vi "Periodic Tasks.vi"(8 "error in":errorcluster) -> ()   [LabVIEW 2020]
doc: "This VI runs in parallel to other tasks. It can contain as many user-defined periodic loops as you need. These can carry out PID or other sorts of timed response."
uses:
  <vilib>/Rock Robotics/WPI/Utilities/WPI_GetSetVariantRefNum.vi
  Robot Global Data.vi
panel:
  out "Limit Switch":bool
  out "Inverted 4":bool
  out "Inverted 3":bool
  out "Inverted 2":bool
  out "Inverted":bool
  out "Right High":dbl
  out "Left High":dbl
  out "Right Low":dbl format="%#_6f"
  out "Left Low":dbl
  out "Arm Red":dbl
  out "Arm Blue2":dbl
  out "Arm Blue":dbl
  out "Fused Heading":dbl
  out "Heading":dbl
  out "Pitch":dbl
  out "Roll":dbl
  out "Calculated yaw":dbl
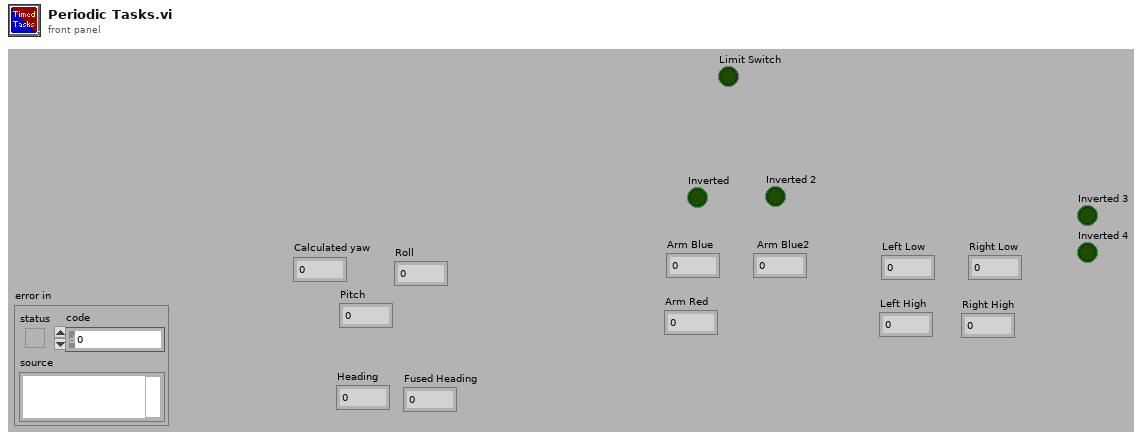
[diagram p1: front panel]
types:
  T1 = typedef "WPI_RobotDriveDevRef.ctl" = cluster{"DevStatus":errorcluster, "Motors[]":T2[], "Square Inputs":bool, "Max Output":dbl}
  T2 = typedef "WPI_MotorControlDeviceRef.ctl" = cluster{"DeviceStatus":errorcluster, "Type":T3, "PWM":cluster{"PWM Channel":T4, "DeadBand":T5}, "CAN":cluster{"Device Number":u8, "SetOutput VI Ref":variant, "GetOutput VI Ref":variant, "Enable VI Ref":variant, "Disable VI Ref":variant, "Data":variant}, "Invert":bool, "DIO PWM":cluster{"PWM \"Enable\" Channel":T4, "DIOChannel":T6, "PWM Rate":dbl}}
  T3 = typedef "WPI_MotorControlType.ctl" = enum16{"PWM", "CAN", "DIO PWM"}
  T4 = typedef "FPGA_DIOPWMChannel.ctl" = enum8{"PWM 0", "PWM 1", "PWM 2", "PWM 3", "PWM 4", "PWM 5", "PWM 6", "PWM 7", "PWM 8", "PWM 9", "PWM MXP 0", "PWM MXP 1", "PWM MXP 2", "PWM MXP 3", "PWM MXP 4", "PWM MXP 5", "PWM MXP 6", "PWM MXP 7", "PWM MXP 8", "PWM MXP 9", "Invalid"}
  T5 = typedef "WPI_PWMDeadband.ctl" = cluster{"Name":string, "maxPositivePwm":i32, "minPositivePwm":i32, "centerPwm":i32, "maxNegativePwm":i32, "minNegativePwm":i32, "angularRange":u16}
  T6 = typedef "FPGA_DIOChannel.ctl" = enum8{"DIO 0", "DIO 1", "DIO 2", "DIO 3", "DIO 4", "DIO 5", "DIO 6", "DIO 7", "DIO 8", "DIO 9", "DIO MXP 0", "DIO MXP 1", "DIO MXP 2", "DIO MXP 3", "DIO MXP 4", "DIO MXP 5", "DIO MXP 6", "DIO MXP 7", "DIO MXP 8", "DIO MXP 9", "DIO MXP 10", "DIO MXP 11", "DIO MXP 12", "DIO MXP 13", "DIO MXP 14", "DIO MXP 15", "SPI Port CS1", "SPI Port CS2", "SPI Port CS3", "SPI Port MISO", "SPI Port MOSI", "Invalid"}
  T7 = typedef "WPI_JoystickDevRef.ctl" = cluster{"Device":T8}
  T8 = typedef "WPI_JoystickDeviceEnum.ctl" = enum16{"USB 0", "USB 1", "USB 2", "USB 3", "USB 4", "USB 5"}
  T9 = cluster{"Motors[][0]":T2, "Motors[][1]":T2, "Motors[][2]":T2, "Motors[][3]":T2, "Motors[][4]":T2, "Motors[][5]":T2, "Motors[][6]":T2, "Motors[][7]":T2, "Motors[][8]":T2}
  T10 = cluster{"JoystickDevRef":T7, "RobotDriveDevRef":T1}
  T11 = cluster{"Yaw":dbl, "Roll":dbl, "Pitch":dbl, "Heading":dbl, "Fused Heading":dbl}
  T12 = typedef "WPI_DigitalInputDevRef.ctl" = cluster{"DevStatus":errorcluster, "DIO Channel":T6}
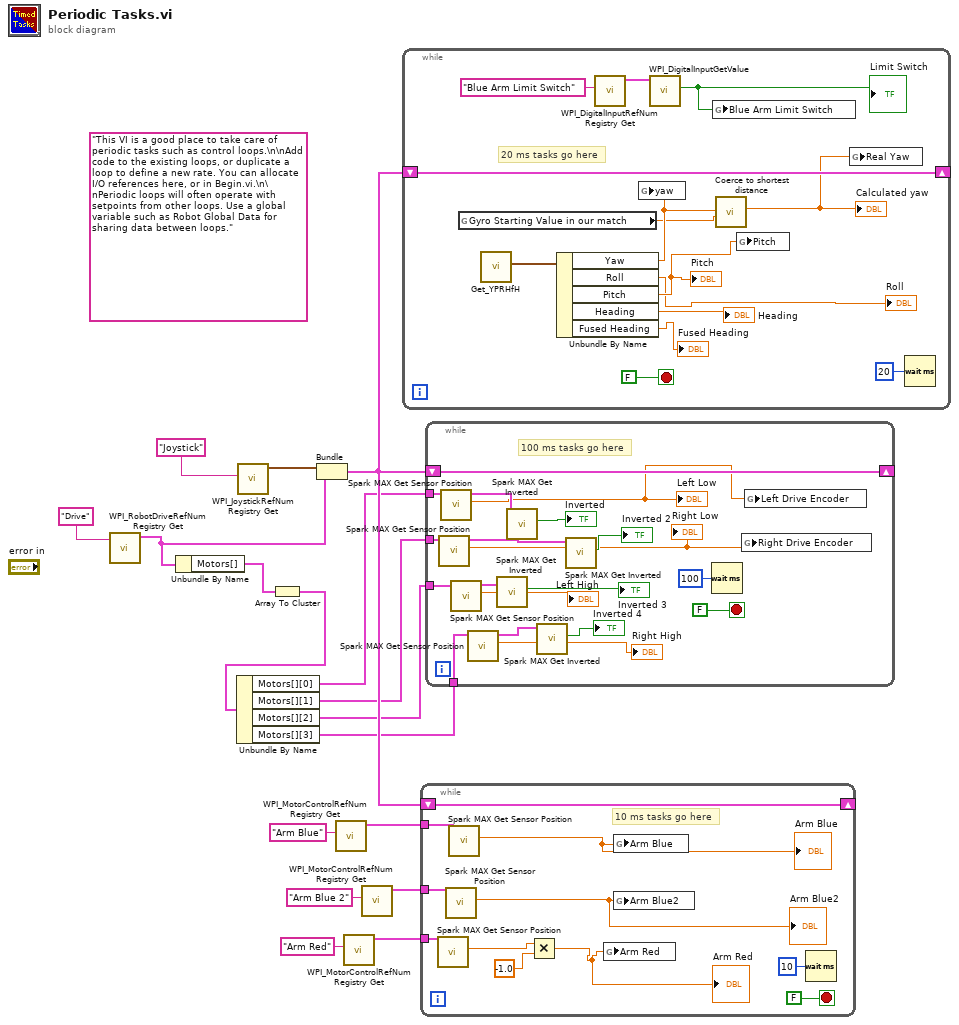
[diagram p0: block diagram]
diagram:
  (unwired) "This VI is a good place to take care of periodic tasks such as control loops.\n\nAdd code to the existing loops, or duplicate a loop to define a new rate. You can allocate I/O references here, or in Begin.vi.\n\nPeriodic loops will often operate with setpoints from other loops. Use a global variable such as Robot Global Data for sharing data between loops."
  n1 = call <vilib>:"WPI_RobotDriveRefNum Registry Get.vi"("refnum name"="Drive") -> ("RobotDriveDevRef"=w1:T1)  [unwired: 1 in, 9 out]
  n2 = Unbundle By Name(w1) -> ("Motors[]"=w8:T2[])
  n3 = call <vilib>:"WPI_JoystickRefNum Registry Get.vi"("refnum name"="Joystick") -> ("JoystickDevRef"=w16:T7)  [unwired: 1 in, 9 out]
  n4 = Array To Cluster(array=w8) -> (cluster=w7:T9)
  n5 = Unbundle By Name(w7) -> ("Motors[][0]"=w6:T2, "Motors[][1]"=w5:T2, "Motors[][2]"=w4:T2, "Motors[][3]"=w3:T2)
  n6 = Bundle("JoystickDevRef"=w16, "RobotDriveDevRef"=w1) -> (w15:T10)  [unwired: 1 out]
  n7 = call <vilib>:"WPI_MotorControlRefNum Registry Get.vi"("refnum name"="Arm Blue") -> ("MotorControlDevRef"=w14:T2)  [unwired: 9 in, 1 out]
  n8 = call <vilib>:"WPI_MotorControlRefNum Registry Get.vi"("refnum name"="Arm Red") -> ("MotorControlDevRef"=w9:T2)  [unwired: 9 in, 1 out]
  n9 = call <vilib>:"WPI_MotorControlRefNum Registry Get.vi"("refnum name"="Arm Blue 2") -> ("MotorControlDevRef"=w10:T2)  [unwired: 9 in, 1 out]
  n10 = while {
    shift-right: [w29] -> _
    shift-left: w15 -> [w29]
    stop <- FALSE stop-if-true
    # "20 ms tasks go here"
    n11 = global read "Robot Global Data.vi" "Gyro Starting Value in our match"() -> (w19:dbl)
    n12 = call <vilib>:"Get_YPRHfH.vi"() -> ("YRPHfH"=w28:T11)  [unwired: 11 in]
    n13 = Unbundle By Name(w28) -> ("Yaw"=w20:dbl, "Roll"=→"Roll":dbl, "Pitch"=w22:dbl, "Heading"=→"Heading":dbl, "Fused Heading"=→"Fused Heading":dbl)
    "Pitch" <- w22
    n14 = call <vilib>:"WPI_DigitalInputRefNum Registry Get.vi"("refnum name"="Blue Arm Limit Switch") -> ("DigitalInputDevRef"=w25:T12)  [unwired: 9 in, 1 out]
    n15 = global write "Robot Global Data.vi" "yaw"(w20) -> ()
    n16 = call <vilib>:"WPI_DigitalInputGetValue.vi"("DigitalInputDevRef"=w25) -> ("Value"=w23:bool)  [unwired: 8 in, 2 out]
    "Limit Switch" <- w23
    n17 = global write "Robot Global Data.vi" "Blue Arm Limit Switch"(w23) -> ()
    n18 = call "Coerce to shortest distance.vi"("Angle 2"=w19, "Angle 1"=w20) -> ("Shortest distance"=w18:dbl)  [unwired: 9 in]
    "Calculated yaw" <- w18
    n19 = global write "Robot Global Data.vi" "Pitch"(w22) -> ()
    n20 = global write "Robot Global Data.vi" "Real Yaw"(w18) -> ()
    n21 = Wait (ms)(milliseconds to wait=u32 20) -> ()  [unwired: 1 out]
  }
  n22 = while {
    shift-right: [w40] -> _
    shift-left: w15 -> [w40]
    tunnel: w14 -> [w39]
    tunnel: w10 -> [w38]
    tunnel: w9 -> [w37]
    stop <- FALSE stop-if-true
    # "10 ms tasks go here"
    n23 = call <vilib>:"Spark MAX Get Sensor Position.vi"("MotorControlDevRef in"=w37) -> ("Sensor Position"=w34:dbl)  [unwired: 7 in, 3 out]
    n24 = call <vilib>:"Spark MAX Get Sensor Position.vi"("MotorControlDevRef in"=w38) -> ("Sensor Position"=w35:dbl)  [unwired: 7 in, 3 out]
    "Arm Blue2" <- w35
    n25 = call <vilib>:"Spark MAX Get Sensor Position.vi"("MotorControlDevRef in"=w39) -> ("Sensor Position"=w36:dbl)  [unwired: 7 in, 3 out]
    "Arm Blue" <- w36
    n26 = Multiply(x=w34, y=-1.0) -> (x*y=w32:dbl)
    "Arm Red" <- w32
    n27 = global write "Robot Global Data.vi" "Arm Red"(w32) -> ()
    n28 = global write "Robot Global Data.vi" "Arm Blue"(w36) -> ()
    n29 = global write "Robot Global Data.vi" "Arm Blue2"(w35) -> ()
    n30 = Wait (ms)(milliseconds to wait=u32 10) -> ()  [unwired: 1 out]
  }
  n31 = while {
    shift-right: [w59] -> _
    shift-left: w15 -> [w59]
    tunnel: w6 -> [w58]
    tunnel: w5 -> [w57]
    tunnel: w4 -> [w56]
    tunnel: w3 -> [w55]
    stop <- FALSE stop-if-true
    # "100 ms tasks go here"
    n32 = call <vilib>:"Spark MAX Get Sensor Position.vi"("MotorControlDevRef in"=w57) -> ("Sensor Position"=w43:dbl, "MotorControlDevRef out"=w50:T2)  [unwired: 7 in, 2 out]
    "Right Low" <- w43
    n33 = call <vilib>:"Spark MAX Get Sensor Position.vi"("MotorControlDevRef in"=w58) -> ("Sensor Position"=w44:dbl, "MotorControlDevRef out"=w52:T2)  [unwired: 7 in, 2 out]
    "Left Low" <- w44
    n34 = call <vilib>:"Spark MAX Get Sensor Position.vi"("MotorControlDevRef in"=w56) -> ("Sensor Position"=→"Left High":dbl, "MotorControlDevRef out"=w48:T2)  [unwired: 7 in, 2 out]
    n35 = call <vilib>:"Spark MAX Get Sensor Position.vi"("MotorControlDevRef in"=w55) -> ("Sensor Position"=→"Right High":dbl, "MotorControlDevRef out"=w46:T2)  [unwired: 7 in, 2 out]
    n36 = call <vilib>:"Spark MAX Get Inverted.vi"("MotorControlDeviceRef in"=w48) -> ("Inverted"=→"Inverted 3":bool)  [unwired: 8 in, 2 out]
    n37 = call <vilib>:"Spark MAX Get Inverted.vi"("MotorControlDeviceRef in"=w52) -> ("Inverted"=→"Inverted":bool)  [unwired: 8 in, 2 out]
    n38 = call <vilib>:"Spark MAX Get Inverted.vi"("MotorControlDeviceRef in"=w46) -> ("Inverted"=→"Inverted 4":bool)  [unwired: 8 in, 2 out]
    n39 = call <vilib>:"Spark MAX Get Inverted.vi"("MotorControlDeviceRef in"=w50) -> ("Inverted"=→"Inverted 2":bool)  [unwired: 8 in, 2 out]
    n40 = Wait (ms)(milliseconds to wait=u32 100) -> ()  [unwired: 1 out]
    n41 = global write "Robot Global Data.vi" "Right Drive Encoder"(w43) -> ()
    n42 = global write "Robot Global Data.vi" "Left Drive Encoder"(w44) -> ()
  }
